vi "julian date of interest.vi"(10 "Day of the year":dbl, 11 "Year":dbl) -> (2 "Julian date of the day":dbl, 3 "Julian date of interest":dbl)   [LabVIEW 2015]
panel:
  out "Fraction of the day":dbl format="%#_13g"
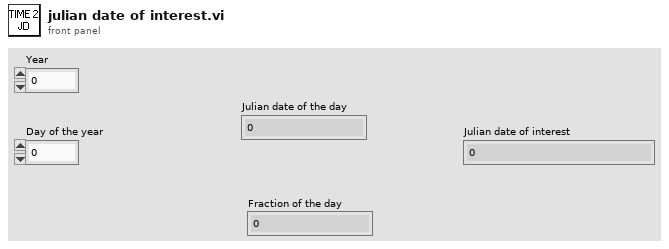
[diagram p1: front panel]
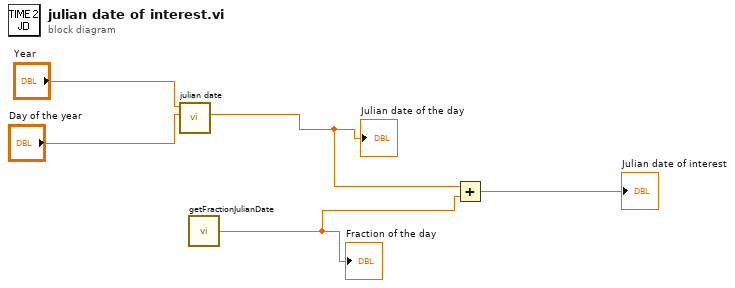
[diagram p0: block diagram]
diagram:
  n1 = call "julian date.vi"("Day of the year"="Day of the year", "Year"="Year") -> ("Julian date of the day"=w3:dbl)  [unwired: 8 in, 1 out]
  "Julian date of the day" <- w3
  n2 = call "getFractionJulianDate.vi"() -> ("Fraction of the day"=w1:dbl)  [unwired: 1 in]
  "Fraction of the day" <- w1
  n3 = Add(x=w3, y=w1) -> (x+y=→"Julian date of interest":dbl)
